vi "Force Accuracy Test DAA.vi"(8 "error in (no error)":errorcluster, 10 "Model in":refnum<class "Model.lvclass">, 11 "Test Actuator State in":refnum<class "Test Actuator State.lvclass">) -> (0 "error out":errorcluster, 1 "Pass":bool, 2 "Model out":refnum<class "Model.lvclass">, 3 "Test Actuator State out":refnum<class "Test Actuator State.lvclass">)   [LabVIEW 2016, in "Test Actuator State.lvclass"]
uses:
  Test Actuator State.lvclass
  Model/Model/Model.lvclass
  <vilib>/Platform/TimedLoop/XDataNode/timing_clust.ctl
  <vilib>/Platform/TimedLoop/XDataNode/nitl_modes.ctl
  <vilib>/Platform/TimedLoop/XDataNode/wakeup.ctl
  Typedefs/ActuatorSetPoints.ctl
  Model/Model/Model.lvclass/Model.ctl
  <vilib>/Analysis/5stat.llb/RMS (DBL).vi
  <vilib>/Analysis/baseanly.llb/Mean (DBL).vi
  <vilib>/platform/TimedLoop/XDataNode/XDataNode.xnode
  Model/Waveforms/Waveform/Waveform.lvclass
  Typedefs/FAMT Typedefs.lvlib
  <vilib>/Analysis/NI_AALPro.lvlib
  <vilib>/Analysis/NI_AALBase.lvlib
  <vilib>/Platform/TimedLoop/XDataNode/XDNodeRunTimeDep.lvlib
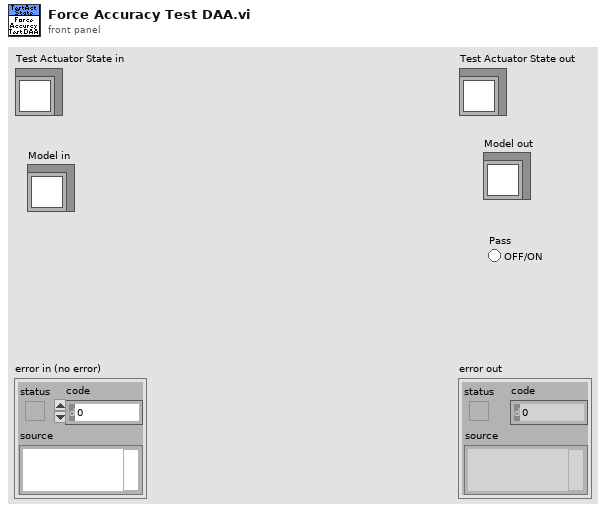
[diagram p1: front panel]
types:
  T1 = typedef "FAMT Typedefs.lvlib/ForceAccuracyTestSettings.ctl" = cluster{"Repeating Error (N)":dbl, "Max Moment (NM)":dbl, "Process Time (s)":dbl, "Sample Time (s)":dbl, "Iterations":i32, "Amplitude (N)":dbl, "Non-Repeating Error":dbl, "Sec Force Error (N)":dbl}
  T2 = typedef "XDNodeRunTimeDep.lvlib/timing_clust.ctl" = cluster{"Expected End [f-1]":u64, "Actual End [f-1]":u64, "Finished Late? [f-1]":bool, "Expected End [i-1]":u64, "Actual End [i-1]":u64, "Finished Late? [i-1]":bool, "Expected Start [i]":u64, "Actual Start [i]":u64, "Expected Start [f]":u64, "Actual Start [f]":u64, "Source Name":string, "Structure Name":string, "Period":i64, "Deadline":i64, "Offset":i64, "Start":i64, "Priority":i32, "Timeout":i32, "Mode":T3, "Wakeup Reason":T4, "Error":errorcluster, "Source Type":string, "Secondary Source Type":string, "Global End Time":u64, "Global Start Time":u64, "Frame Duration":u64, "Iteration Duration":u64, "Assigned CPU":i32, "I/O Scan Engine Mode":u32}
  T3 = typedef "XDNodeRunTimeDep.lvlib/nitl_modes.ctl" = enum32{"No Change", "Process missed periods, maintain original phase", "Discard missed periods, maintain original phase", "Process missed periods, ignore original phase", "Discard missed periods, ignore original phase"}
  T4 = typedef "XDNodeRunTimeDep.lvlib/wakeup.ctl" = enum32{"Normal", "Aborted", "Asynchronous wakeup", "Timing source error", "Timed loop error", "Timeout"}
  T5 = typedef "FAMT Typedefs.lvlib/ActuatorSetPoints.ctl" = cluster{"Axial Force":dbl, "Lateral Force":dbl, "FC1 Force":dbl, "FC2 Force":dbl}
  T6 = typedef "FAMT Typedefs.lvlib/ActuatorData.ctl" = cluster{"Timestamp":dbl, "Axial Force":dbl, "Lateral Force":dbl, "FC1 Force":dbl, "FC2 Force":dbl, "Lateral Push Pressure":dbl, "Lateral Pull Pressure":dbl, "Axial Push Pressure":dbl, "Axial Pull Pressure":dbl}
  T7 = typedef "FAMT Typedefs.lvlib/ToveyEngData.ctl" = cluster{"Timestamp":dbl, "Fx":dbl, "Fy":dbl, "Fz":dbl, "Mx":dbl, "My":dbl, "Mz":dbl}
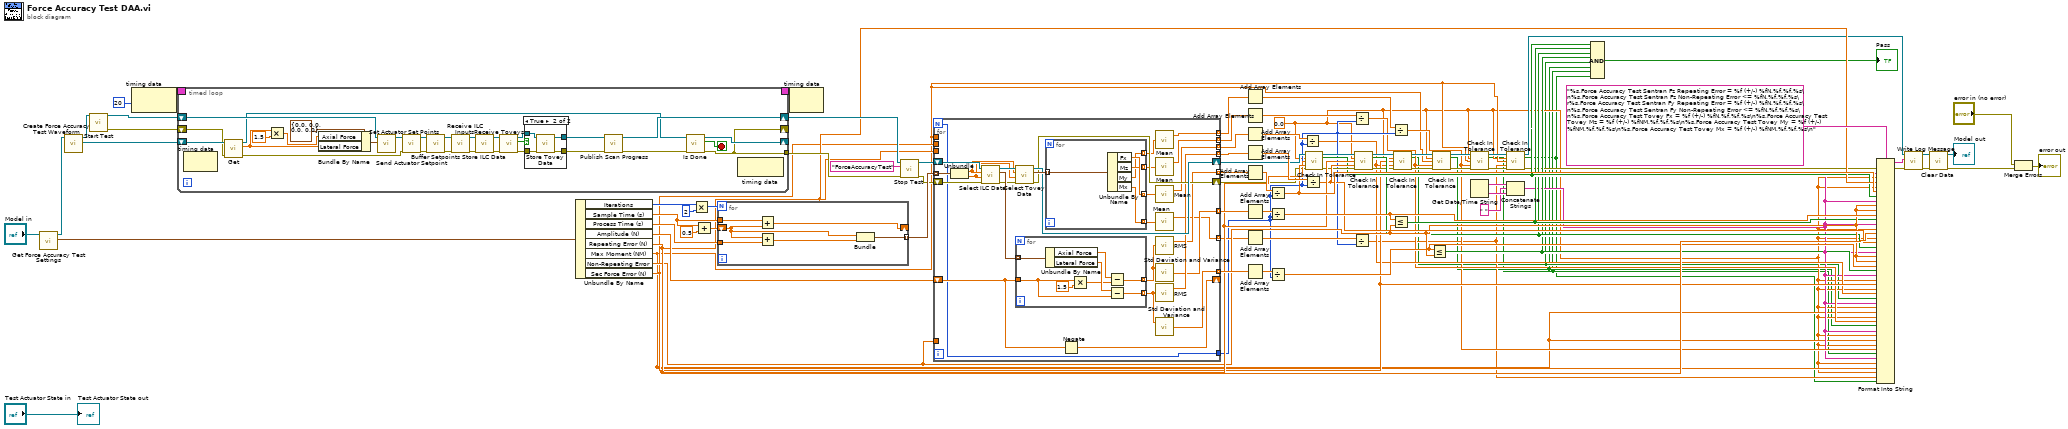
[diagram p0: block diagram]
diagram:
  w6 = 0.0 ("Expected")
  n1 = call-dynamic "Get Force Accuracy Test Settings.vi"("Model in"="Model in") -> ("Force Accuracy Test Settings"=w86:T1, "Model out"=w87:refnum<class "Model.lvclass">)  [unwired: 9 in]
  n2 = call "Create Force Accuracy Test Waveform.vi"("Model in"=w87) -> ("Waveform"=w83:refnum<class "Waveform.lvclass">, "Model out"=w73:refnum<class "Model.lvclass">)  [unwired: 9 in]
  n3 = call "Start Test.vi"("Model in"=w73) -> ("error out"=w71:errorcluster, "Model out"=w72:refnum<class "Model.lvclass">)  [unwired: 9 in]
  n4 = node-c288(i64 20 ("Period")) -> (w76:T2)
  n5 = timed-loop {
    shift-right: [w118] -> w67
    shift-left: w72 -> [w110]
    shift-right: [w92] -> _
    shift-left: w71 -> [w104]
    shift-right: [w100] -> _
    shift-left: w83 -> [w106]
    timing: w76 -> [_]
    timing-out: [_] -> w75
    tunnel: [w92] -> w64
    stop <- w101 stop-if-true
    n6 = node-c288() -> ()  [unwired: 1 in, 1 out]
    n7 = call-dynamic "Get.vi"("error in (no error)"=w104, "Waveform in"=w106) -> ("error out"=w103:errorcluster, "Value"=w99:dbl, "Waveform out"=w105:refnum<class "Waveform.lvclass">)  [unwired: 7 in]
    n8 = Multiply(x=w99, y=1.5) -> (x*y=w97:dbl)
    n9 = Bundle By Name(cluster=T5 {"Axial Force"=0.0, "Lateral Force"=0.0, "FC1 Force"=0.0, "FC2 Force"=0.0} ("Actuator Set Points"), "Axial Force"=w97, "Lateral Force"=w99) -> (w107:T5)
    n10 = call "Set Actuator Set Points.vi"("Actuator Set Points"=w107, "Model in"=w110) -> ("Model out"=w109:refnum<class "Model.lvclass">)  [unwired: 9 in]
    n11 = call "Send Actuator Setpoint.vi"("error in (no error)"=w103, "Model in"=w109) -> ("error out"=w94:errorcluster, "Model out"=w96:refnum<class "Model.lvclass">)  [unwired: 8 in]
    n12 = call "Buffer Setpoints.vi"("error in (no error)"=w94, "Model in"=w96) -> ("error out"=w93:errorcluster, "Model out"=w95:refnum<class "Model.lvclass">)  [unwired: 8 in]
    n13 = call "Receive ILC Inputs.vi"("error in (no error)"=w93, "Model in"=w95) -> ("error out"=w119:errorcluster, "Model out"=w120:refnum<class "Model.lvclass">)  [unwired: 8 in]
    n14 = call "Store ILC Data.vi"("error in (no error)"=w119, "Model in"=w120) -> ("error out"=w116:errorcluster, "Model out"=w117:refnum<class "Model.lvclass">)  [unwired: 8 in]
    n15 = call "Receive Toveys.vi"("error in (no error)"=w116, "Model in"=w117) -> ("error out"=w114:errorcluster, "Data Received"=w113:bool, "Model out"=w115:refnum<class "Model.lvclass">)  [unwired: 7 in]
    n16 = case shown="True" w113 {
      tunnel: w115 -> [w124 w128]
      tunnel: w114 -> [w123 w127]
      tunnel: [w123 w126] -> w111
      tunnel: [w124 w125] -> w112
      frame False {
      }
      frame True {
        n17 = call "Store Tovey Data.vi"("error in (no error)"=w127, "Model in"=w128) -> ("error out"=w126:errorcluster, "Model out"=w125:refnum<class "Model.lvclass">)  [unwired: 8 in]
      }
    }
    n18 = call "Publish Scan Progress.vi"("error in (no error)"=w111, "Model in"=w112) -> ("error out"=w102:errorcluster, "Model out"=w118:refnum<class "Model.lvclass">)  [unwired: 8 in]
    n19 = call-dynamic "Is Done.vi"("error in (no error)"=w102, "Waveform in"=w105) -> ("error out"=w92:errorcluster, "Is Done"=w101:bool, "Waveform out"=w100:refnum<class "Waveform.lvclass">)  [unwired: 7 in]
    n20 = node-c288() -> ()  [unwired: 1 in, 1 out]
  }
  n21 = Unbundle By Name(w86) -> ("Iterations"=w70:i32, "Sample Time (s)"=w79:dbl, "Process Time (s)"=w80:dbl, "Amplitude (N)"=w77:dbl, "Repeating Error (N)"=w51:dbl, "Max Moment (NM)"=w7:dbl, "Non-Repeating Error"=w49:dbl, "Sec Force Error (N)"=w12:dbl)
  n22 = Multiply(x=w70, y=2) -> (x*y=w68:i32)
  n23 = Add(x=w79, y=0.5) -> (x+y=w81:dbl)
  n24 = for {
    N: w68 -> [_]
    shift-right: [w132] -> _
    shift-left: w81 -> [w130]
    tunnel: w80 -> [w134]
    tunnel: w79 -> [w133]
    tunnel: [w129] -> w78 mode=indexing
    n25 = Add(x=w133, y=w130) -> (x+y=w132:dbl)
    n26 = Add(x=w130, y=w134) -> (x+y=w131:dbl)
    n27 = Bundle(w130, w131) -> (w129:cluster{dbl, dbl})  [unwired: 1 in]
  }
  n28 = node-c288(w75) -> ()  [unwired: 1 out]
  n29 = call "Stop Test.vi"("error in (no error)"=w64, "Test"="ForceAccuracyTest", "Model in"=w67) -> ("error out"=w63:errorcluster, "Model out"=w65:refnum<class "Model.lvclass">)  [unwired: 7 in]
  n30 = for {
    N -> [w139]
    tunnel: w78 -> [w162] mode=indexing
    shift-right: [w152] -> w44
    shift-left: w65 -> [w161]
    shift-right: [w159] -> _
    shift-left: w77 -> [w150]
    shift-right: [w151] -> w40
    shift-left: w63 -> [w158]
    tunnel: w51 -> [_]
    tunnel: w7 -> [_]
    tunnel: w49 -> [_]
    tunnel: w12 -> [_]
    tunnel: [w143] -> w61 mode=indexing
    tunnel: [w142] -> w59 mode=indexing
    tunnel: [w141] -> w57 mode=indexing
    tunnel: [w140] -> w56 mode=indexing
    tunnel: [w139] -> w23
    tunnel: [w138] -> w31 mode=indexing
    tunnel: [w137] -> w30 mode=indexing
    tunnel: [w136] -> w29 mode=indexing
    tunnel: [w135] -> w28 mode=indexing
    n31 = Unbundle(w162) -> (w156:dbl, w155:dbl)
    n32 = call "Select ILC Data.vi"("error in (no error)"=w158, "End Time"=w155, "Start Time"=w156, "Model in"=w161) -> ("error out"=w154:errorcluster, "Data"=w160:T6[], "Model out"=w157:refnum<class "Model.lvclass">)  [unwired: 4 in, 1 out]
    n33 = call "Select Tovey Data.vi"("error in (no error)"=w154, "End Time"=w155, "Start Time"=w156, "Model in"=w157) -> ("error out"=w151:errorcluster, "Data"=w153:T7[], "Model out"=w152:refnum<class "Model.lvclass">)  [unwired: 4 in, 1 out]
    n34 = for {
      tunnel: w160 -> [w175] mode=indexing
      tunnel: w150 -> [w170]
      tunnel: [w174] -> w145 mode=indexing
      tunnel: [w172] -> w144 mode=indexing
      n35 = Unbundle By Name(w175) -> ("Axial Force"=w171:dbl, "Lateral Force"=w173:dbl)
      n36 = Multiply(x=w170, y=1.5) -> (x*y=w168:dbl)
      n37 = Subtract(x=w171, y=w168) -> (x-y=w174:dbl)
      n38 = Subtract(x=w173, y=w170) -> (x-y=w172:dbl)
    }
    n39 = for {
      tunnel: [w167] -> w149 mode=indexing
      tunnel: [w166] -> w148 mode=indexing
      tunnel: [w165] -> w147 mode=indexing
      tunnel: [w164] -> w146 mode=indexing
      tunnel: w153 -> [w163] mode=indexing
      n40 = Unbundle By Name(w163) -> ("Fx"=w167:dbl, "Mz"=w166:dbl, "My"=w165:dbl, "Mx"=w164:dbl)
    }
    n41 = Negate(x=w150) -> (-x=w159:dbl)
    n42 = call-poly <vilib>:"Mean.vi"("X"=w147) -> ("mean"=w136:dbl)  [unwired: 1 out]
    n43 = call-poly <vilib>:"Mean.vi"("X"=w148) -> ("mean"=w137:dbl)  [unwired: 1 out]
    n44 = call-poly <vilib>:"Mean.vi"("X"=w149) -> ("mean"=w138:dbl)  [unwired: 1 out]
    n45 = call-poly <vilib>:"Mean.vi"("X"=w146) -> ("mean"=w135:dbl)  [unwired: 1 out]
    n46 = call-poly <vilib>:"RMS.vi"("X"=w145) -> ("rms value"=w141:dbl)  [unwired: 1 out]
    n47 = call <vilib>:"Std Deviation and Variance.vi"("X"=w145) -> ("standard deviation"=w140:dbl)  [unwired: 1 in, 2 out]
    n48 = call-poly <vilib>:"RMS.vi"("X"=w144) -> ("rms value"=w143:dbl)  [unwired: 1 out]
    n49 = call <vilib>:"Std Deviation and Variance.vi"("X"=w144) -> ("standard deviation"=w142:dbl)  [unwired: 1 in, 2 out]
  }
  n50 = Add Array Elements(numeric array=w29) -> (sum=w27:dbl)
  n51 = Add Array Elements(numeric array=w30) -> (sum=w25:dbl)
  n52 = Add Array Elements(numeric array=w31) -> (sum=w24:dbl)
  n53 = Add Array Elements(numeric array=w61) -> (sum=w62:dbl)
  n54 = Add Array Elements(numeric array=w57) -> (sum=w58:dbl)
  n55 = Add Array Elements(numeric array=w56) -> (sum=w55:dbl)
  n56 = Add Array Elements(numeric array=w28) -> (sum=w26:dbl)
  n57 = Add Array Elements(numeric array=w59) -> (sum=w60:dbl)
  n58 = Divide(x=w58, y=w23) -> (x/y=w53:dbl)
  n59 = Divide(x=w55, y=w23) -> (x/y=w52:dbl)
  n60 = Divide(x=w60, y=w23) -> (x/y=w48:dbl)
  n61 = Divide(x=w24, y=w23) -> (x/y=w11:dbl)
  n62 = Divide(x=w62, y=w23) -> (x/y=w50:dbl)
  n63 = call "Check In Tolerance.vi"("Model in"=w44, "Expected"=w6, "Tolerance"=w51, "Actual"=w53, "error in (no error)"=w40) -> ("Model out"=w43:refnum<class "Model.lvclass">, "Pass"=w36:bool, "error out"=w39:errorcluster)  [unwired: 8 in]
  n64 = Divide(x=w25, y=w23) -> (x/y=w10:dbl)
  n65 = Divide(x=w26, y=w23) -> (x/y=w5:dbl)
  n66 = call "Check In Tolerance.vi"("Model in"=w43, "Expected"=w6, "Tolerance"=w51, "Actual"=w50, "error in (no error)"=w39) -> ("Model out"=w17:refnum<class "Model.lvclass">, "Pass"=w34:bool, "error out"=w22:errorcluster)  [unwired: 8 in]
  n67 = Divide(x=w27, y=w23) -> (x/y=w9:dbl)
  n68 = Less Or Equal?(x=w52, y=w49) -> (x <= y?=w35:bool)
  n69 = call "Check In Tolerance.vi"("Model in"=w17, "Expected"=w6, "Tolerance"=w12, "Actual"=w11, "error in (no error)"=w22) -> ("Model out"=w16:refnum<class "Model.lvclass">, "Pass"=w4:bool, "error out"=w21:errorcluster)  [unwired: 8 in]
  n70 = Less Or Equal?(x=w48, y=w49) -> (x <= y?=w33:bool)
  n71 = call "Check In Tolerance.vi"("Model in"=w16, "Expected"=w6, "Tolerance"=w7, "Actual"=w10, "error in (no error)"=w21) -> ("Model out"=w15:refnum<class "Model.lvclass">, "Pass"=w3:bool, "error out"=w20:errorcluster)  [unwired: 8 in]
  n72 = call "Check In Tolerance.vi"("Model in"=w15, "Expected"=w6, "Tolerance"=w7, "Actual"=w9, "error in (no error)"=w20) -> ("Model out"=w14:refnum<class "Model.lvclass">, "Pass"=w2:bool, "error out"=w19:errorcluster)  [unwired: 8 in]
  n73 = Get Date/Time String() -> (date string=w47:string, time string=w46:string)  [unwired: 3 in]
  n74 = call "Check In Tolerance.vi"("Model in"=w14, "Expected"=w6, "Tolerance"=w7, "Actual"=w5, "error in (no error)"=w19) -> ("Model out"=w13:refnum<class "Model.lvclass">, "Pass"=w1:bool, "error out"=w18:errorcluster)  [unwired: 8 in]
  n75 = Concatenate Strings(w47, " " ("string"), w46) -> (w8:string)
  n76 = Compound Arithmetic op=AND(w36, w35, w34, w33, w4, w3, w2, w1) -> (→"Pass":bool)
  n77 = Format Into String(format string="%s,Force Accuracy Test Sentran Fz Repeating Error = %f (+/-) %fN,%f,%f,%s\n%s,Force Accuracy Test Sentran Fz Non-Repeating Error <= %fN,%f,%f,%s\r%s,Force Accuracy Test Sentran Fy Repeating Error = %f (+/-) %fN,%f,%f,%s\n%s,Force Accuracy Test Sentran Fy Non-Repeating Error <= %fN,%f,%f,%s\n%s,Force Accuracy Test Tovey Fx = %f (+/-) %fN,%f,%f,%s\n%s,Force Accuracy Test Tovey Mz = %f (+/-) %fNM,%f,%f,%s\n%s,Force Accuracy Test Tovey My = %f (+/-) %fNM,%f,%f,%s\n%s,Force Accuracy Test Tovey Mx = %f (+/-) %fNM,%f,%f,%s\n", error in=w18, w8, w6, w51, w6, w53, w36, w8, w49, w49, w52, w35, w8, w6, w51, w6, w50, w34, w8, w49, w49, w48, w33, w8, w6, w12, w6, w11, w4, w8, w6, w7, w6, w10, w3, w8, w6, w7, w6, w9, w2, w8, w6, w7, w6, w5, w1) -> (resulting string=w41:string, error out=w38:errorcluster)  [unwired: 1 in]
  n78 = call "Write Log Message.vi"("error in (no error)"=w38, "Message"=w41, "Model in"=w13) -> ("error out"=w37:errorcluster, "Model out"=w42:refnum<class "Model.lvclass">)  [unwired: 7 in]
  n79 = call "Clear Data.vi"("error in (no error)"=w37, "Model in"=w42) -> ("error out"=w85:errorcluster, "Model out"=→"Model out":refnum<class "Model.lvclass">)  [unwired: 8 in]
  n80 = Merge Errors("error in (no error)", w85) -> (→"error out":errorcluster)
  "Test Actuator State out" <- "Test Actuator State in"
